vi "GetChannelBoardType.vi"(8 "error in (no error)":errorcluster, 9 "Parameters":T2, 10 "Channel":u8, 11 "ConnectionID IN":i32) -> (0 "error out":errorcluster, 1 "Fichier .ecc":string, 2 "BoardType":T1(ring), 3 "ConnectionID Out":i32)   [LabVIEW 2022 SP3, in "EClib functions.lvlib"]
uses:
  EClib functions.lvlib
  Parameters.ctl
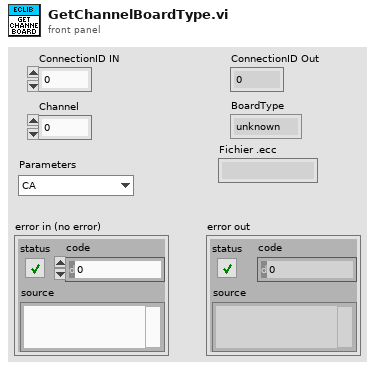
[diagram p1: front panel]
types:
  T1 = enum16{"unknown", "essential", "premium", "premium digicore"}
  T2 = typedef "EClib functions.lvlib/Parameters.ctl" = enum16{"CA", "CASG", "CP", "GEIS", "ISCAN", "OCV", "PEIS", "SCCX", "SGEIS", "SPEIS", "VSCAN", "MP"}
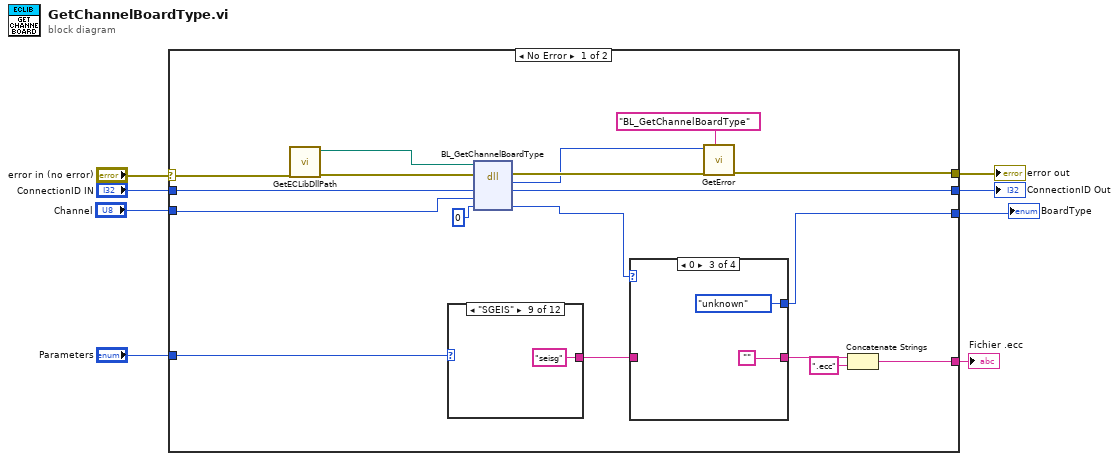
[diagram p0: block diagram]
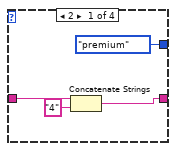
[diagram p2: hidden frame]
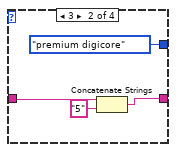
[diagram p3: hidden frame]
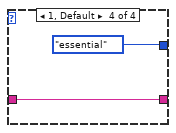
[diagram p4: hidden frame]
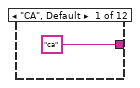
[diagram p5: hidden frame]
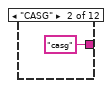
[diagram p6: hidden frame]
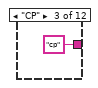
[diagram p7: hidden frame]
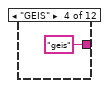
[diagram p8: hidden frame]
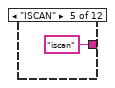
[diagram p9: hidden frame]
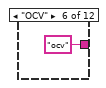
[diagram p10: hidden frame]
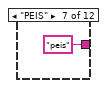
[diagram p11: hidden frame]
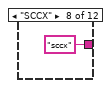
[diagram p12: hidden frame]
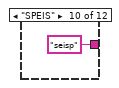
[diagram p13: hidden frame]
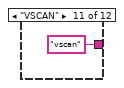
[diagram p14: hidden frame]
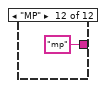
[diagram p15: hidden frame]
diagram:
  n1 = case shown="No Error" "error in (no error)" {
    selector: "error in (no error)" -> [w23 w52]
    tunnel: [w18 w52] -> w8
    tunnel: [w9 _] -> w1
    tunnel: "Channel" -> [w24 _]
    tunnel: "ConnectionID IN" -> [w26 w51]
    tunnel: [w16 w51] -> w4
    tunnel: "Parameters" -> [w15 _]
    tunnel: [w11 _] -> w2
    frame No Error {
      n2 = call "GetECLibDllPath.vi"("error in (no error)"=w23) -> ("error out"=w22:errorcluster, "ECLibDLLPath"=w21:path)  [unwired: 9 in]
      n3 = case shown="\"SGEIS\"" w15 {
        tunnel: ["ca" "casg" "cp" "geis" "iscan" "ocv" "peis" "sccx" "seisg" "seisp" "vscan" "mp"] -> w14
        frame "CA", Default {
        }
        frame "CASG" {
        }
        frame "CP" {
        }
        frame "GEIS" {
        }
        frame "ISCAN" {
        }
        frame "OCV" {
        }
        frame "PEIS" {
        }
        frame "SCCX" {
        }
        frame "SGEIS" {
        }
        frame "SPEIS" {
        }
        frame "VSCAN" {
        }
        frame "MP" {
        }
      }
      n4 = dll-call lib="?" fn="BL_GetChannelBoardType"(path in=w21, error in=w22, "ConnectionID"=w26, "Channel"=w24, "ChannelType"=u32 0) -> (error out=w19:errorcluster, "return type"=w17:i32, "ConnectionID"=w16:i32, "ChannelType"=w10:u32)  [unwired: 2 in, 1 out]
      n5 = case shown="0" w10 {
        tunnel: w14 -> [w30 w33 _ w38]
        tunnel: [w28 w32 "" w38] -> w13
        tunnel: [T1."premium" ("BoardType") T1."premium digicore" ("BoardType") T1."unknown" ("BoardType") T1."essential" ("BoardType")] -> w9
        frame 2 {
          n6 = Concatenate Strings(w30, "4" ("string")) -> (w28:string)
        }
        frame 3 {
          n7 = Concatenate Strings(w33, "5" ("string")) -> (w32:string)
        }
        frame 0 {
        }
        frame 1, Default {
        }
      }
      n8 = call "GetError.vi"("DLLFunction"="BL_GetChannelBoardType", "error in"=w19, "code"=w17) -> ("error out"=w18:errorcluster)  [unwired: 8 in]
      n9 = Concatenate Strings(w13, ".ecc" ("string")) -> (w11:string)
    }
    frame Error {
    }
  }
  "error out" <- w8
  "ConnectionID Out" <- w4
  "Fichier .ecc" <- w2
  "BoardType" <- w1
